vi "Create All Message Queues.vi"(8 "error in (no error)":errorcluster) -> (0 "error out":errorcluster, 3 "Message Queues out":T1)   [LabVIEW 2025, in "Message Queue.lvlib"]
doc: "This VI creates and initializes all the message queues for your application. If your application requires more than one message queue, right-click the \"Message Queues\" constant above and select Open Type Def. Add the new Message Queue(s) to the type definition, then initialize them in this VI."
uses:
  Message Queue.lvlib
  All Message Queues.ctl
  Message Cluster.ctl
  Enqueue Message (Single).vi
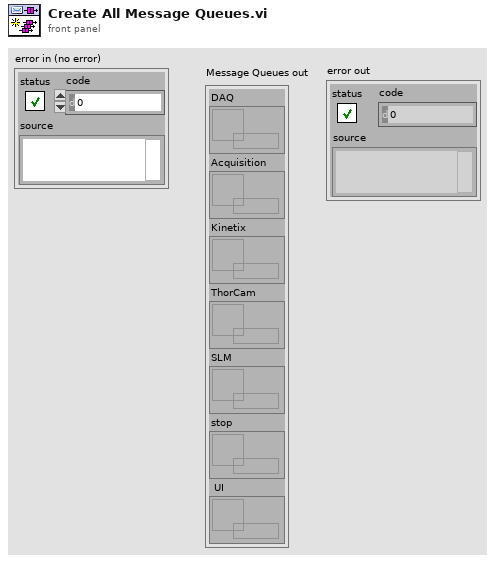
[diagram p1: front panel]
types:
  T1 = typedef "Message Queue.lvlib/All Message Queues.ctl" = cluster{"DAQ":refnum<queue>, "Acquisition":refnum<queue>, "Kinetix":refnum<queue>, "ThorCam":refnum<queue>, "SLM":refnum<queue>, "stop":refnum<queue>, " UI":refnum<queue>}
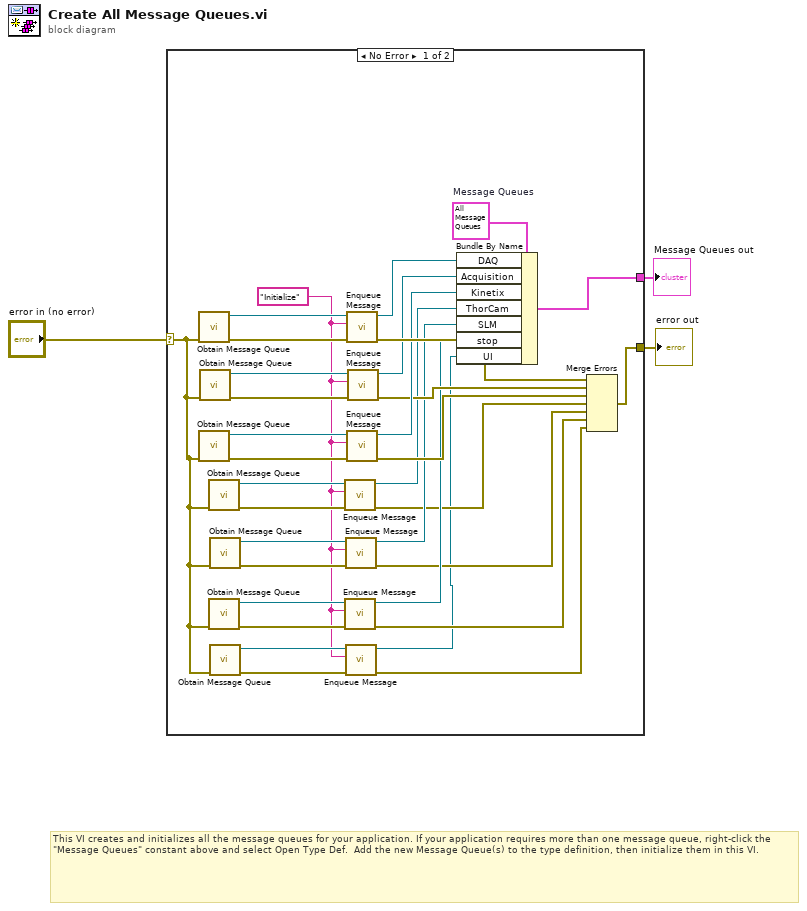
[diagram p0: block diagram]
diagram:
  # "This VI creates and initializes all the message queues for your application. If your application requires more than one message queue, right-click the \"Message Queues\" constant above and select Open Type Def.  Add the new Message Queue(s) to the type definition, then initialize them in this VI."
  n1 = case shown="No Error" "error in (no error)" {
    selector: "error in (no error)" -> [w7 w37]
    tunnel: [w24 w37] -> w3
    tunnel: [w34 _] -> w2
    frame No Error {
      w6 = "Initialize" ("Message")
      w35 = T1 {"DAQ"=refnum, "Acquisition"=refnum, "Kinetix"=refnum, "ThorCam"=refnum, "SLM"=refnum, "stop"=refnum, " UI"=refnum}  # Message Queues
      n2 = call "Obtain Message Queue.vi"("error in (no error)"=w7) -> ("error out"=w33:errorcluster, "Message Queue"=w32:refnum<queue>)  [unwired: 9 in]
      n3 = call "Obtain Message Queue.vi"("error in (no error)"=w7) -> ("error out"=w29:errorcluster, "Message Queue"=w28:refnum<queue>)  [unwired: 9 in]
      n4 = call "Obtain Message Queue.vi"("error in (no error)"=w7) -> ("error out"=w30:errorcluster, "Message Queue"=w31:refnum<queue>)  [unwired: 9 in]
      n5 = call "Obtain Message Queue.vi"("error in (no error)"=w7) -> ("error out"=w19:errorcluster, "Message Queue"=w18:refnum<queue>)  [unwired: 9 in]
      n6 = call "Obtain Message Queue.vi"("error in (no error)"=w7) -> ("error out"=w21:errorcluster, "Message Queue"=w17:refnum<queue>)  [unwired: 9 in]
      n7 = call "Obtain Message Queue.vi"("error in (no error)"=w7) -> ("error out"=w20:errorcluster, "Message Queue"=w16:refnum<queue>)  [unwired: 9 in]
      n8 = call "Obtain Message Queue.vi"("error in (no error)"=w7) -> ("error out"=w9:errorcluster, "Message Queue"=w8:refnum<queue>)  [unwired: 9 in]
      n9 = call-poly "Enqueue Message.vi"("error in (no error)"=w19, "Message"=w6, "Message Queue"=w18) -> ("error out"=w10:errorcluster, "dup Message Queue"=w15:refnum<queue>)  [unwired: 7 in]
      n10 = call-poly "Enqueue Message.vi"("error in (no error)"=w21, "Message"=w6, "Message Queue"=w17) -> ("error out"=w12:errorcluster, "dup Message Queue"=w13:refnum<queue>)  [unwired: 7 in]
      n11 = call-poly "Enqueue Message.vi"("error in (no error)"=w20, "Message"=w6, "Message Queue"=w16) -> ("error out"=w11:errorcluster, "dup Message Queue"=w14:refnum<queue>)  [unwired: 7 in]
      n12 = call-poly "Enqueue Message.vi"("error in (no error)"=w9, "Message"=w6, "Message Queue"=w8) -> ("error out"=w4:errorcluster, "dup Message Queue"=w5:refnum<queue>)  [unwired: 7 in]
      n13 = call-poly "Enqueue Message.vi"("error in (no error)"=w33, "Message"=w6, "Message Queue"=w32) -> ("error out"=w36:errorcluster, "dup Message Queue"=w27:refnum<queue>)  [unwired: 7 in]
      n14 = call-poly "Enqueue Message.vi"("error in (no error)"=w29, "Message"=w6, "Message Queue"=w28) -> ("error out"=w22:errorcluster, "dup Message Queue"=w25:refnum<queue>)  [unwired: 7 in]
      n15 = call-poly "Enqueue Message.vi"("error in (no error)"=w30, "Message"=w6, "Message Queue"=w31) -> ("error out"=w23:errorcluster, "dup Message Queue"=w26:refnum<queue>)  [unwired: 7 in]
      n16 = Bundle By Name(cluster=w35, "DAQ"=w27, "Acquisition"=w26, "Kinetix"=w25, "ThorCam"=w15, "SLM"=w14, "stop"=w13, "UI"=w5) -> (w34:T1)
      n17 = Merge Errors(w36, w23, w22, w10, w11, w12, w4) -> (w24:errorcluster)
    }
    frame Error {
    }
  }
  "Message Queues out" <- w2
  "error out" <- w3
